vi "Version Number.vi"() -> (1 "Version Number":string)   [LabVIEW 2020]
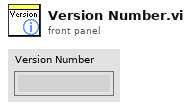
[diagram p1: front panel]
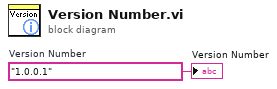
[diagram p0: block diagram]
diagram:
  w1 = "1.0.0.1"  # Version Number
  "Version Number" <- w1
